vi "Reset Signal Configuration.vi"(8 "error in (no error)":errorcluster, 11 "signal configuration in":refnum<class "SV Discrete Sweep.lvclass">) -> (0 "error out":errorcluster, 3 "signal configuration out":refnum<class "SV Discrete Sweep.lvclass">)   [LabVIEW 2017, in "SV Discrete Sweep.lvclass"]
uses:
  <vilib>/addons/_NISVFA/_Generation/Signal Generation/SV Discrete Sweep/SV Discrete Sweep.lvclass
  C:/Program Files (x86)/National Instruments/LabVIEW 2017/vi.lib/addons/_NISVFA/_Generation/Signal Generation/SV Function/SV Function.lvclass
  <vilib>/addons/_NISVFA/_Generation/Signal Generation/SV Discrete Sweep/SV Discrete Sweep.lvclass/SV Discrete Sweep.ctl
  <vilib>/addons/_NISVFA/_Generation/Signal Generation/SV Function/SV Function.lvclass
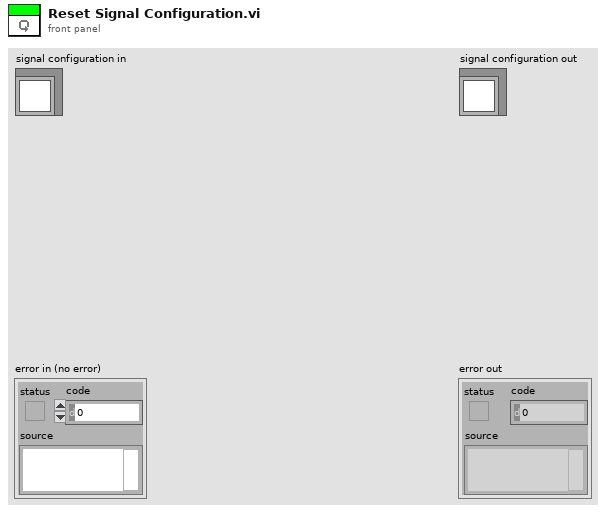
[diagram p1: front panel]
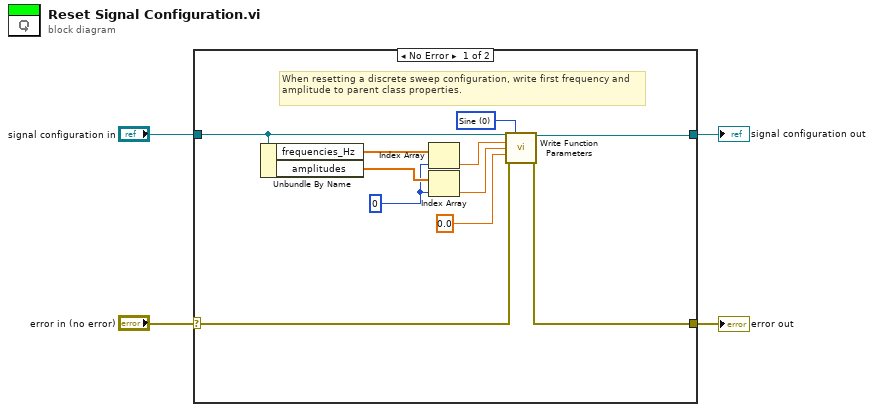
[diagram p0: block diagram]
diagram:
  n1 = case shown="No Error" "error in (no error)" {
    selector: "error in (no error)" -> [w6 w16]
    tunnel: [w5 w16] -> w3
    tunnel: [w8 w17] -> w2
    tunnel: "signal configuration in" -> [w9 w17]
    frame No Error {
      w10 = 0 ("samples")
      w15 = u16 0 items=["Sine", "Triangle", "Square", "Sawtooth"] ("function type")
      # "When resetting a discrete sweep configuration, write first frequency and amplitude to parent class properties."
      n2 = Unbundle By Name(w9) -> ("frequencies_Hz"=w11:dbl[], "amplitudes"=w14:dbl[])
      n3 = Index Array(array=w11, index=w10) -> (element=w13:dbl)
      n4 = Index Array(array=w14, index=w10) -> (element=w12:dbl)
      n5 = call <vilib>:"Write Function Parameters.vi"("signal configuration"=w9, "function type"=w15, "frequency (Hz)"=w13, "amplitude"=w12, "phase (deg)"=0.0, "error in (no error)"=w6) -> ("signal configuration"=w8:refnum<class "SV Discrete Sweep.lvclass">, "error out"=w5:errorcluster)  [unwired: 8 in]
    }
    frame Error {
    }
  }
  "error out" <- w3
  "signal configuration out" <- w2
